vi "Datatypes.vi"() -> ()   [LabVIEW 2012]
panel:
  in  "text control":string
  out "String Indicator":string
  in  "Boolean":bool
  out "Boolean":bool
  out "Float indicator":dbl
  in  "Floating point control":dbl
  out "Integer Indicator":dbl
  in  "Integer control":dbl
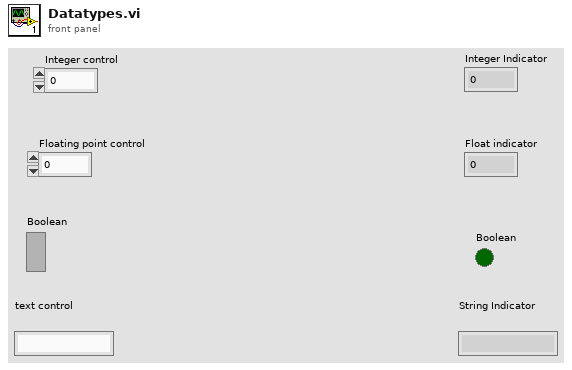
[diagram p1: front panel]
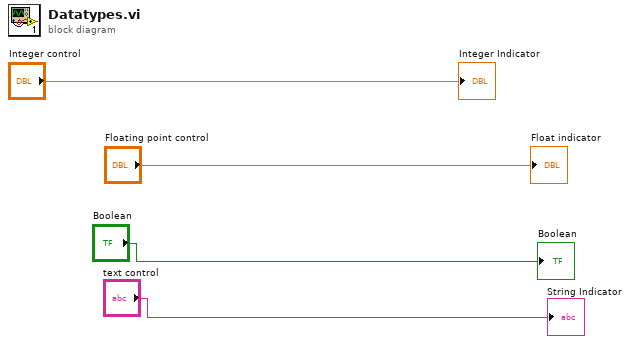
[diagram p0: block diagram]
diagram:
  "Integer Indicator" <- "Integer control"
  "Float indicator" <- "Floating point control"
  "Boolean" <- "Boolean"
  "String Indicator" <- "text control"
